vi "Teste Send instruction.vi"() -> ()   [LabVIEW 2018]
panel:
  out "ms":u32
  out "error out":errorcluster
  out "error":bool
  out "ok":bool
  out "response":string
  in  "instruction":string
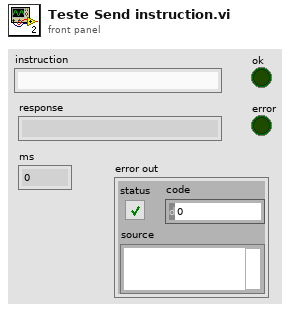
[diagram p1: front panel]
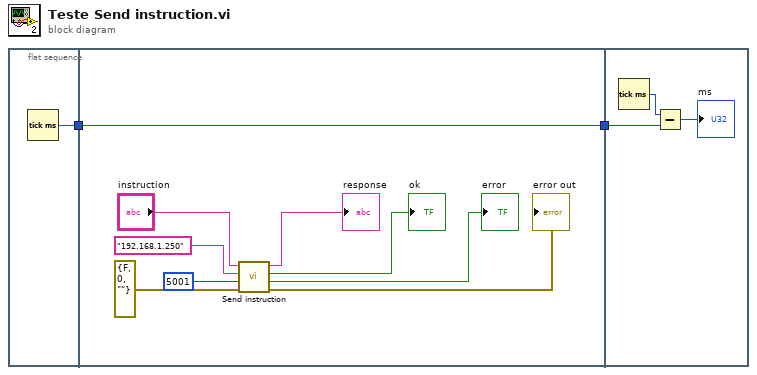
[diagram p0: block diagram]
diagram:
  n1 = flat-sequence {
    tunnel: [w3] -> w1
    tunnel: [w4] -> w2
    tunnel: w1 -> [w4]
    tunnel: w2 -> [w14]
    frame #0 {
      n2 = Tick Count (ms)() -> (millisecond timer value=w3:u32)
    }
    frame #1 {
      n3 = call "Send instruction.vi"("error in (no error)"=errorcluster {"status"=FALSE, "code"=0, "source"=""}, "motor port"=u16 5001, "motor ip"="192.168.1.250", "instruction"="instruction") -> ("error out"=→"error out":errorcluster, "error"=→"error":bool, "ok"=→"ok":bool, "response"=→"response":string)  [unwired: 4 in]
    }
    frame #2 {
      n4 = Tick Count (ms)() -> (millisecond timer value=w15:u32)
      n5 = Subtract(x=w15, y=w14) -> (x-y=→"ms":u32)
    }
  }
